vi "Day09-1.vi"() -> ()   [LabVIEW 2021]
uses:
  e8067021-3399-4566-9da4-0f30890c607a.vi
panel:
  out "sum":i32
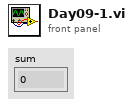
[diagram p1: front panel]
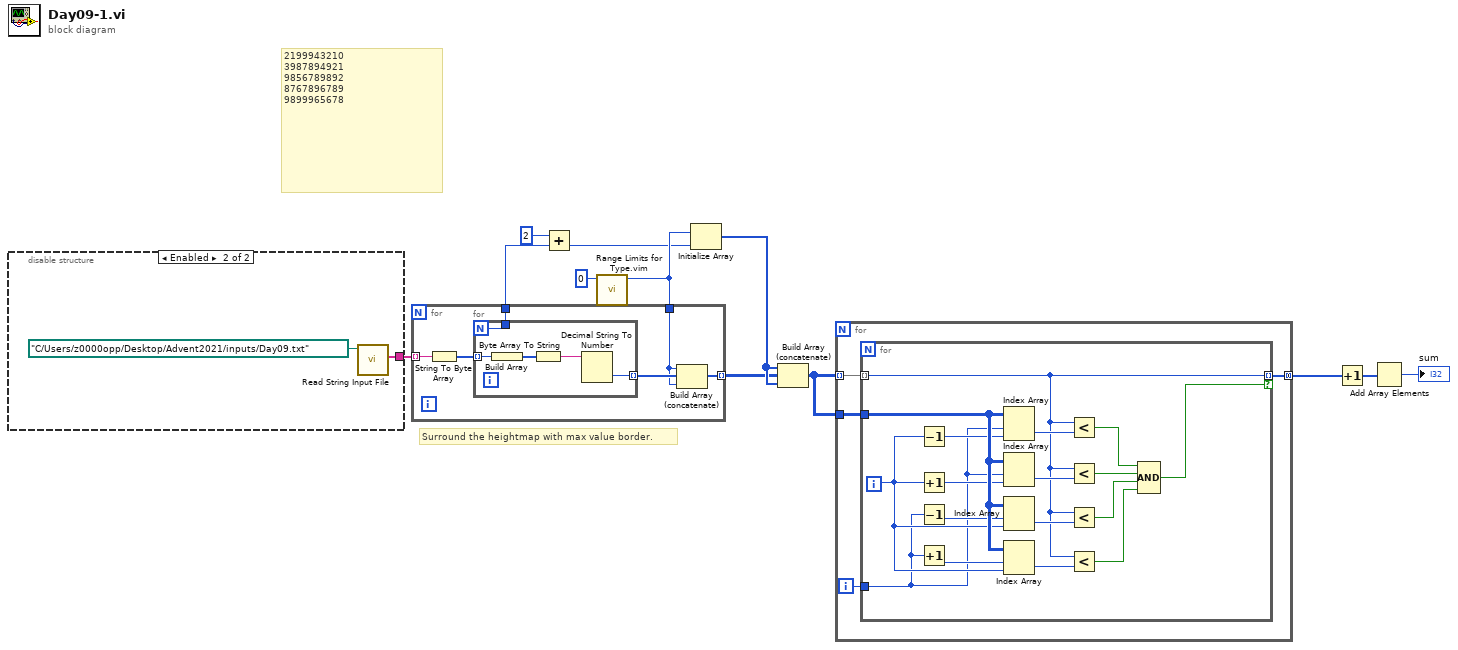
[diagram p0: block diagram]
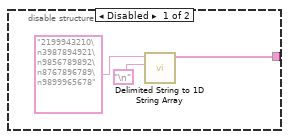
[diagram p2: hidden frame]
diagram:
  # "Surround the heightmap with max value border."
  # "2199943210\n3987894921\n9856789892\n8767896789\n9899965678"
  n1 = disable-structure shown="Enabled" {
    disable-tunnel: [w13 w16] -> w12
    frame Disabled {
      n2 = call <vilib>:"Delimited String to 1D String Array.vi"("delimiter"="\n", "delimited string"="2199943210\n3987894921\n9856789892\n8767896789\n9899965678") -> ("string array"=w13:string[])  [unwired: 9 in]
    }
    frame Enabled {
      n3 = call "Read String Input File.vi"("file path (dialog if empty)"=path "C:/Users/z0000opp/Desktop/Advent2021/inputs/Day09.txt") -> ("input values"=w16:string[])  [unwired: 10 in]
    }
  }
  n4 = call "Range Limits for Type.vim"("type"=0) -> ("maximum value for type"=w10:i32)  [unwired: 9 in, 1 out]
  n5 = for {
    tunnel: w12 -> [w23] mode=indexing
    tunnel: [w19] -> w5 mode=indexing
    tunnel: w10 -> [w20]
    tunnel: [w18] -> w9
    n6 = String To Byte Array(string=w23) -> (unsigned byte array=w22:u8[])
    n7 = for {
      N -> [w24]
      tunnel: w22 -> [w28] mode=indexing
      tunnel: [w25] -> w21 mode=indexing
      tunnel: [w24] -> w18
      n8 = Build Array(w28) -> (w27:u8[])
      n9 = Byte Array To String(unsigned byte array=w27) -> (string=w26:string)
      n10 = Decimal String To Number(string=w26) -> (number=w25:i32)  [unwired: 2 in, 1 out]
    }
    n11 = Build Array (concatenate)(w20, w21, w20) -> (w19:i32[])
  }
  n12 = Add(x=2, y=w9) -> (x+y=w8:i32)
  n13 = Initialize Array(w10, w8) -> (w6:i32[])
  n14 = Build Array (concatenate)(w6, w5, w6) -> (w4:i32[][])
  n15 = for {
    tunnel: w4 -> [w32] mode=indexing
    tunnel: w4 -> [w31]
    tunnel: [w29] -> w3 mode=concatenating
    i -> [w30]
    n16 = for {
      tunnel: w32 -> [w34] mode=indexing
      tunnel: w31 -> [w49]
      tunnel: w30 -> [w43]
      tunnel: [w34] -> w29 mode=indexing if=w33
      i -> [w46]
      n17 = Decrement(x=w46) -> (x-1=w48:i32)
      n18 = Increment(x=w46) -> (x+1=w47:i32)
      n19 = Decrement(x=w43) -> (x-1=w45:i32)
      n20 = Increment(x=w43) -> (x+1=w44:i32)
      n21 = Index Array(array=w49, index (row)=w43, index (col)=w48) -> (element=w42:i32)
      n22 = Index Array(array=w49, index (row)=w43, index (col)=w47) -> (element=w41:i32)
      n23 = Index Array(array=w49, index (row)=w45, index (col)=w46) -> (element=w40:i32)
      n24 = Index Array(array=w49, index (row)=w44, index (col)=w46) -> (element=w39:i32)
      n25 = Less?(x=w34, y=w42) -> (x < y?=w38:bool)
      n26 = Less?(x=w34, y=w41) -> (x < y?=w37:bool)
      n27 = Less?(x=w34, y=w40) -> (x < y?=w36:bool)
      n28 = Less?(x=w34, y=w39) -> (x < y?=w35:bool)
      n29 = Compound Arithmetic op=AND(w38, w37, w36, w35) -> (w33:bool)
    }
  }
  n30 = Increment(x=w3) -> (x+1=w1:i32[])
  n31 = Add Array Elements(numeric array=w1) -> (sum=→"sum":i32)
